vi "LVIS_VerifyStrLen.vi"(7 "Field Name":string, 8 "Error In":errorcluster, 10 "Max StrLen":i32, 11 "Field Value In":string) -> (0 "Error Out":errorcluster)   [LabVIEW 2015]
doc: "Verifies the field value for a given field name is valid, else throws an error."
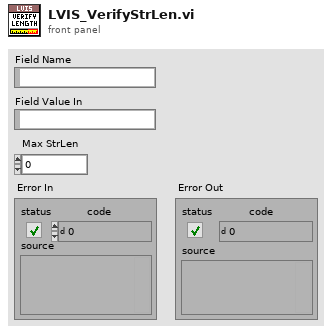
[diagram p1: front panel]
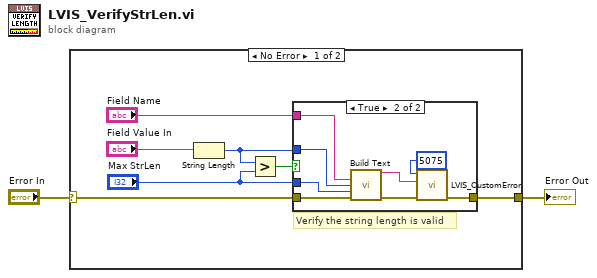
[diagram p0: block diagram]
diagram:
  n1 = case shown="No Error" "Error In" {
    selector: "Error In" -> [w9 w19]
    tunnel: [w8 w19] -> w1
    frame No Error {
      # "Verify the string length is valid"
      n2 = String Length(string="Field Value In") -> (length=w4:i32)
      n3 = Greater?(x=w4, y="Max StrLen") -> (0:w6:bool)
      n4 = case shown="True" w6 {
        tunnel: w9 -> [w10 w16]
        tunnel: [w10 w17] -> w8
        tunnel: "Field Name" -> [_ w13]
        tunnel: w4 -> [_ w12]
        tunnel: "Max StrLen" -> [_ w11]
        frame False {
        }
        frame True {
          n5 = call "Build Text"("Field"=w13, "Act"=w12, "Max"=w11, "error in (no error)"=w16) -> ("Result"=w14:string, "error out"=w15:errorcluster)  [unwired: 10 in]
          n6 = call "LVIS_CustomError.vi"("error in (no error)"=w15, "Addiitional Info"=w14, "Code"=5075) -> ("error out"=w17:errorcluster)  [unwired: 8 in]
        }
      }
    }
    frame Error {
    }
  }
  "Error Out" <- w1
